vi "main_jgxu_double.vi"() -> ()   [LabVIEW 2012]
panel:
  out "Current-Time":cluster{dbl[], dbl[]}[](graph)
  in  "Quit":bool
  out "Voltage-Current":cluster{dbl[], dbl[]}[](graph)
  in  "Mode":enum32{"Main Panel", "0254 Initialize"}(tab)
  out "Boolean 2":bool
  in  "Start_2400":bool
  out "Time (s)":dbl
  in  "Delay (ms)":u32=1000
  in  "Target (V)":dbl=0.01
  in  "Step (V)":dbl=0.001
  in  "Stop":bool
  in  "file path (use dialog)":path=path "D:/TD/20171116/5-3/test.txt"
  in  "Ch1 Set":dbl=0.01
  out "Ch1 PV":dbl
  in  "Set Ch1":bool
  out "Boolean":bool
  out "SV_CH1":dbl
  in  "Ch2 Set Set":dbl=0.01
  out "SV_CH2":dbl
  out "Ch2 PV":dbl
  in  "Set Ch2":bool
  in  "VISA 2400":refnum<visa-resource-name>
  in  "VISA 0254":refnum<visa-resource-name>
  in  "Gas Flow Enable":bool
  in  "VISA 2450":refnum<visa-resource-name>
  in  "Target (V) Plas":dbl=0.01
  in  "Step (V) Plas":dbl=0.001
  in  "Initialization":bool
  out "Initiliazation Started":bool
  # "sccm"
  # "sccm"
  # "sccm"
  # "sccm"
  # "sccm"
  # "sccm"
  # "Please Wait  ~ 25 s"
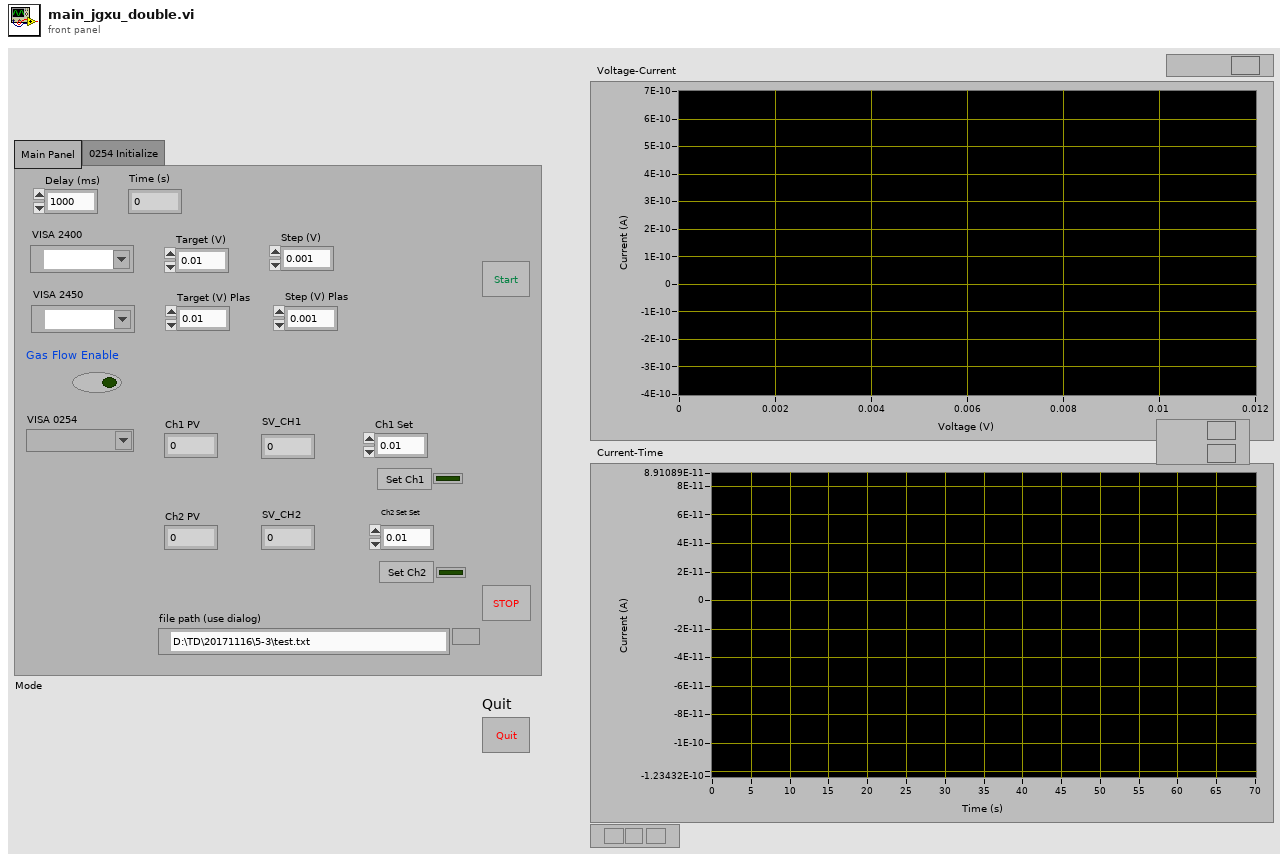
[diagram p1: front panel]
types:
  T1 = enum16{"open", "replace", "create", "open or create", "replace or create", "replace or create with confirmation"}
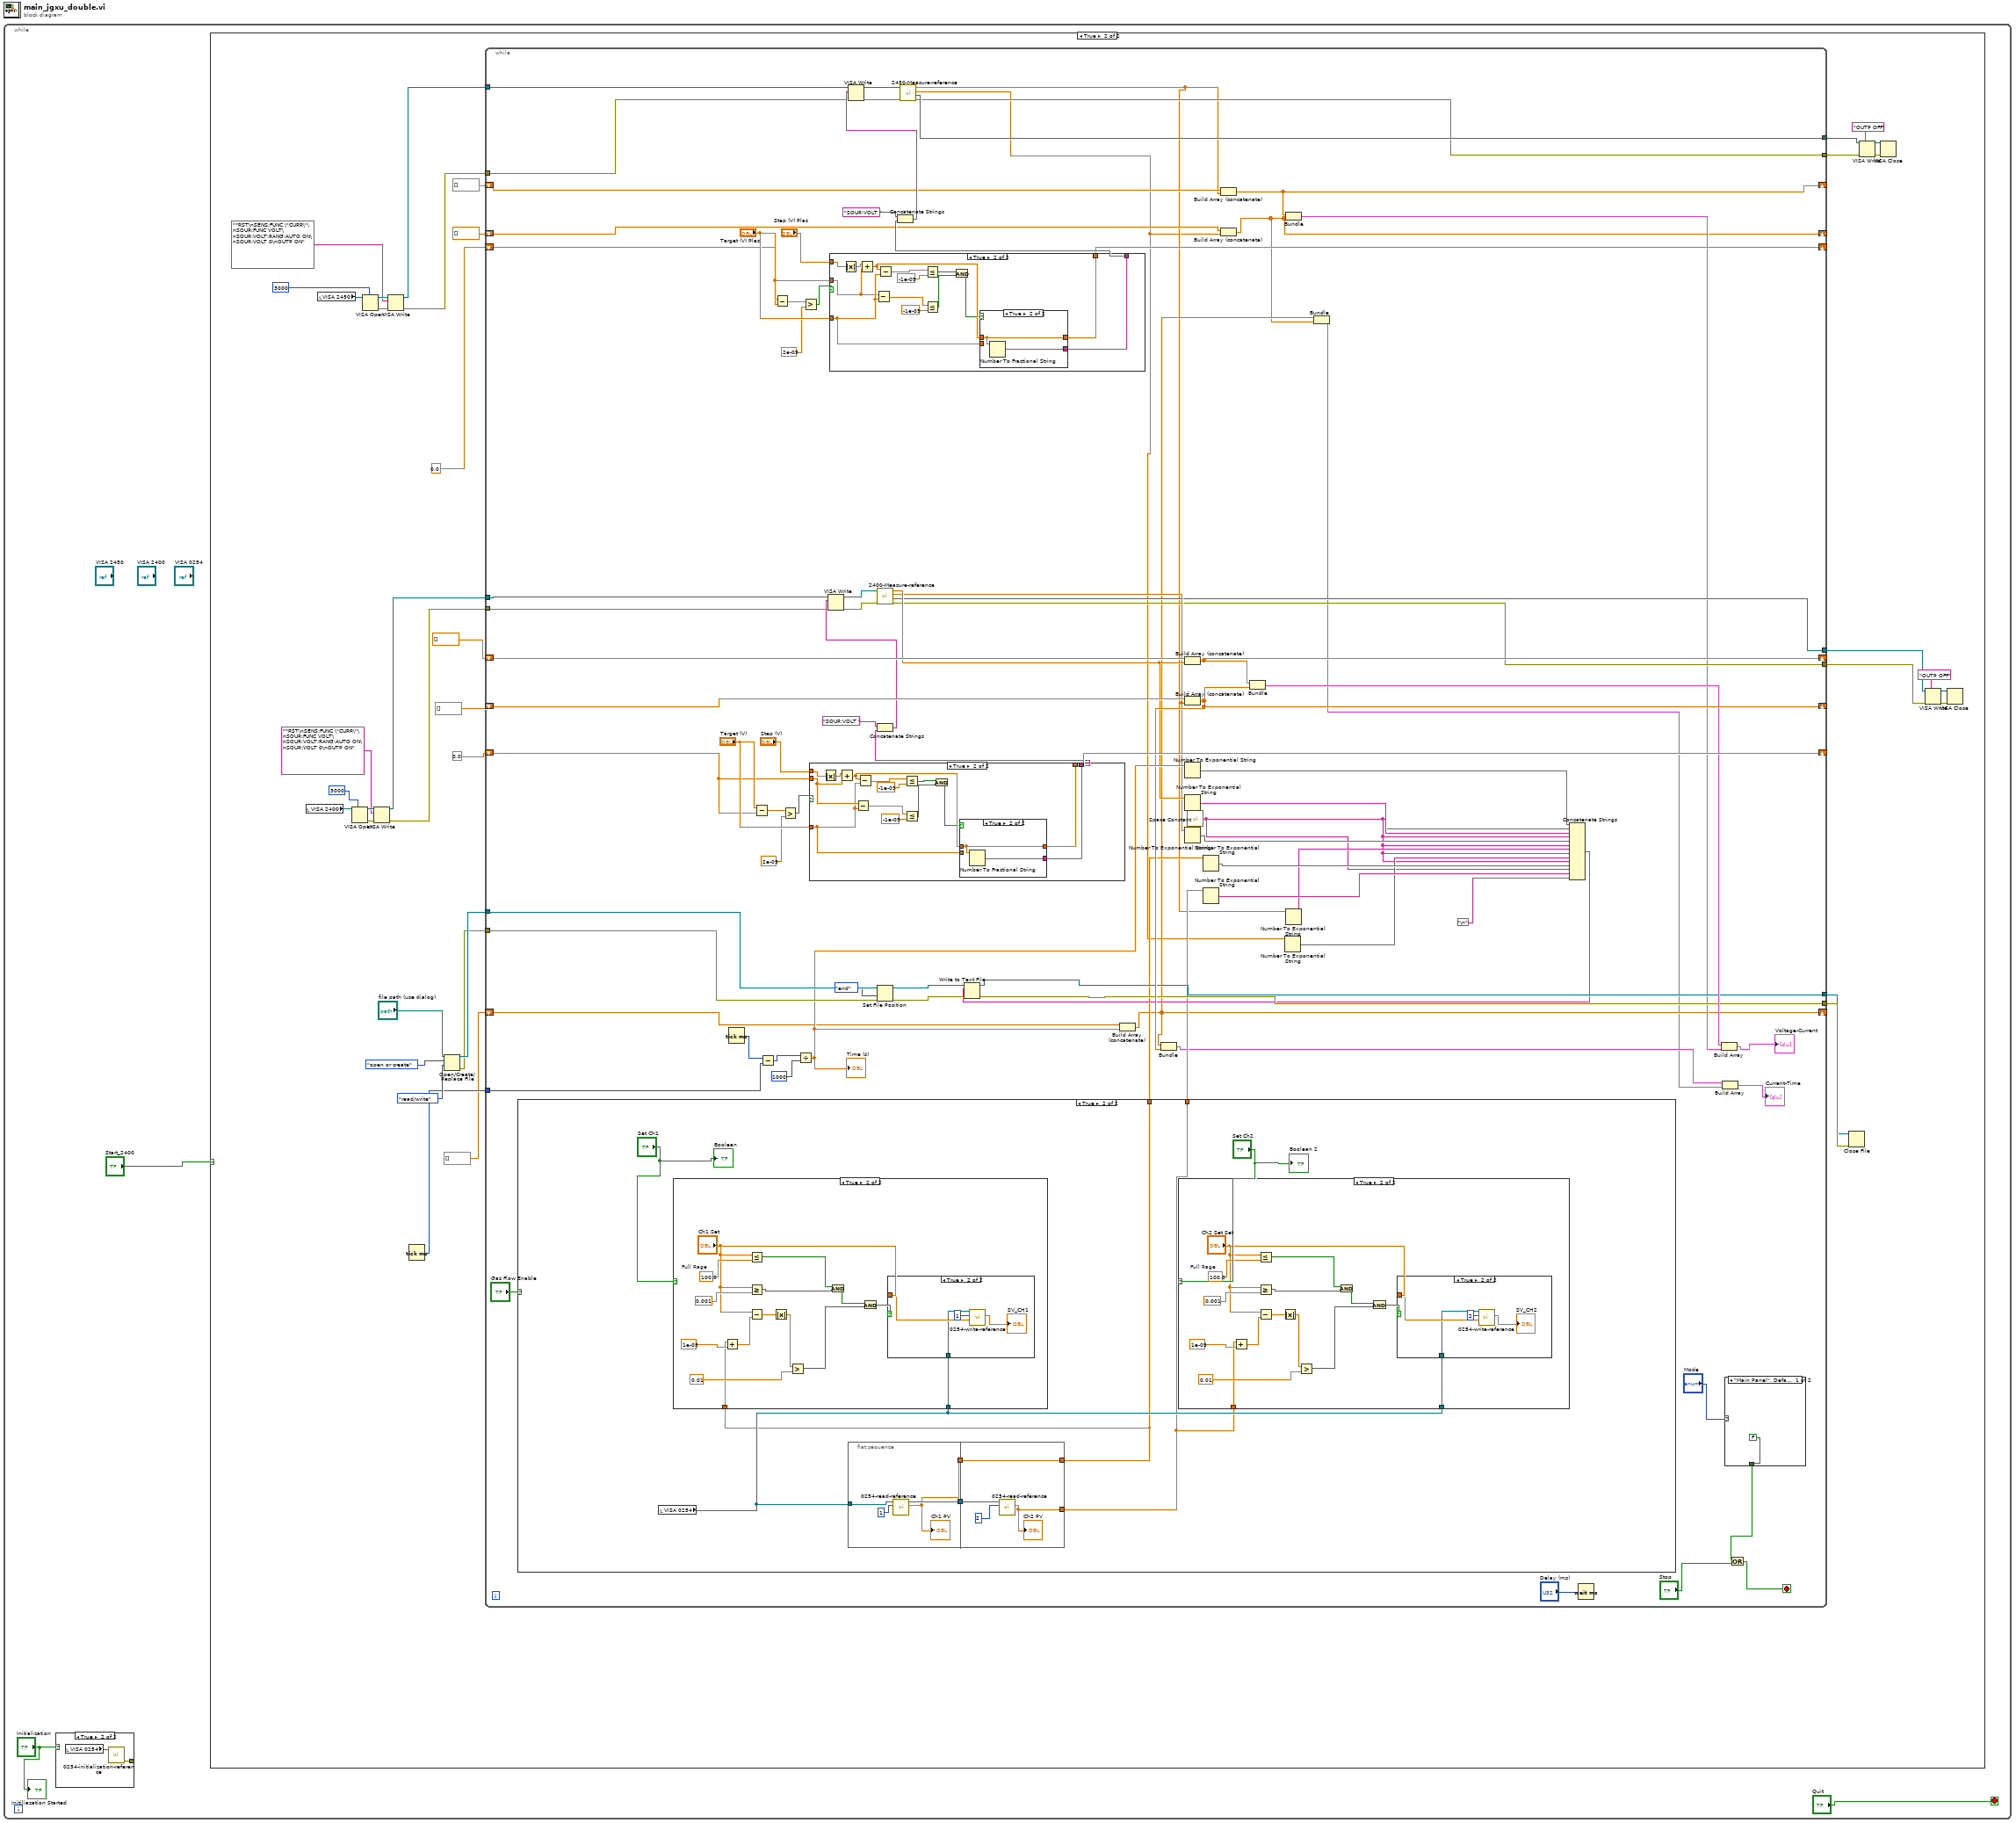
[diagram p0: block diagram]
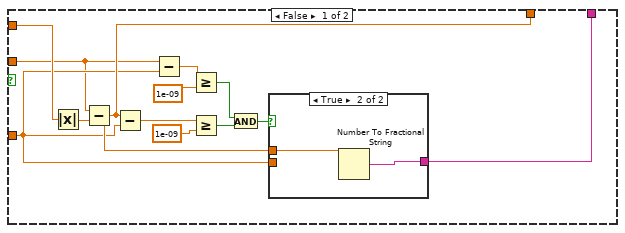
[diagram p3: hidden frame]
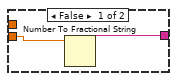
[diagram p4: hidden frame]
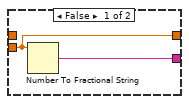
[diagram p5: hidden frame]
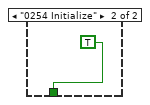
[diagram p6: hidden frame]
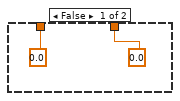
[diagram p7: hidden frame]
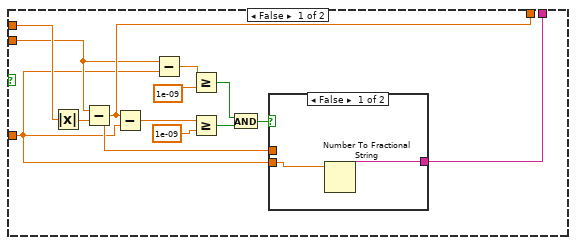
[diagram p12: hidden frame]
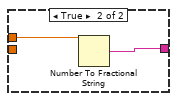
[diagram p13: hidden frame]
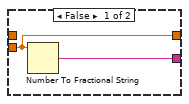
[diagram p14: hidden frame]
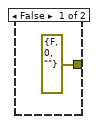
[diagram p15: hidden frame]
diagram:
  n1 = while {
    stop <- "Quit" stop-if-true
    n2 = case shown="True" "Initialization" {
      tunnel: [errorcluster {"status"=FALSE, "code"=0, "source"=""} ("error out") w253] -> _
      frame False {
      }
      frame True {
        n3 = local read "VISA 0254"() -> (w254:refnum<visa-resource-name>)
        n4 = call "0254-initialization-reference.vi"("0254-VISA"=w254) -> ("error out"=w253:errorcluster)  [unwired: 8 in, 2 out]
      }
    }
    n5 = case shown="True" "Start_2400" {
      frame False {
      }
      frame True {
        n6 = local read "VISA 2400"() -> (w28:refnum<visa-resource-name>)
        n7 = local read "VISA 2450"() -> (w15:refnum<visa-resource-name>)
        n8 = VISA Open(timeout (0)=3000 ("timeout ms (488.2 global)"), VISA resource name=w28) -> (VISA resource name=w31:refnum<visa-resource-name>, error out=w30:errorcluster)  [unwired: 3 in]
        n9 = VISA Open(timeout (0)=3000 ("timeout ms (488.2 global)"), VISA resource name=w15) -> (VISA resource name=w18:refnum<visa-resource-name>, error out=w17:errorcluster)  [unwired: 3 in]
        n10 = VISA Write(VISA resource name=w31, write buffer="*RST\nSENS:FUNC \"CURR\"\nSOUR:FUNC VOLT\nSOUR:VOLT:RANG:AUTO ON\nSOUR:VOLT 0\nOUTP ON" ("data"), error in (no error)=w30) -> (VISA resource name out=w25:refnum<visa-resource-name>, error out=w26:errorcluster)  [unwired: 1 out]
        n11 = VISA Write(VISA resource name=w18, write buffer="*RST\nSENS:FUNC \"CURR\"\nSOUR:FUNC VOLT\nSOUR:VOLT:RANG:AUTO ON\nSOUR:VOLT 0\nOUTP ON" ("data"), error in (no error)=w17) -> (VISA resource name out=w13:refnum<visa-resource-name>, error out=w12:errorcluster)  [unwired: 1 out]
        n12 = Tick Count (ms)() -> (millisecond timer value=w33:u32)
        n13 = Open/Create/Replace File(file path (use dialog)="file path (use dialog)", operation (0:open)=T1."open or create", access (0:read/write)=enum16{"read/write", "read-only", "write-only"}."read/write") -> (refnum out=w38:refnum<file>, error out=w37:errorcluster)  [unwired: 1 in, 3 out]
        n14 = while {
          shift-right: [w111] -> _
          shift-left: 0.0 ("Target (V)") -> [w107]
          shift-right: [w120] -> _
          shift-left: dbl[] [] -> [w123]
          shift-right: [w95] -> _
          shift-left: dbl[] [] -> [w122]
          tunnel: w38 -> [w117]
          tunnel: w37 -> [w116]
          tunnel: [w90] -> w36
          tunnel: [w91] -> w35
          tunnel: w25 -> [w103]
          tunnel: [w82] -> w21
          tunnel: [w81] -> w20
          tunnel: w26 -> [w94]
          tunnel: w33 -> [w101]
          shift-right: [w53] -> _
          shift-left: dbl[] [] -> [w96]
          tunnel: w13 -> [w65]
          tunnel: w12 -> [w64]
          shift-right: [w62] -> _
          shift-left: 0.0 ("Target (V)") -> [w63]
          tunnel: [w61] -> w7
          tunnel: [w60] -> w6
          shift-right: [w56] -> _
          shift-left: dbl[] [] -> [w57]
          shift-right: [w52] -> _
          shift-left: dbl[] [] -> [w55]
          stop <- w76 stop-if-true
          n15 = case shown="True" "Gas Flow Enable" {
            tunnel: [0.0 ("PV") w165] -> w88
            tunnel: [0.0 ("PV") w164] -> w87
            frame False {
            }
            frame True {
              n16 = local read "VISA 0254"() -> (w169:refnum<visa-resource-name>)
              n17 = case shown="True" "Set Ch1" {
                tunnel: w169 -> [_ w199]
                tunnel: w165 -> [_ w198]
                frame False {
                }
                frame True {
                  w202 = 100.0  # Full Rage
                  n18 = Add(x=w198, y=1e-05) -> (x+y=w211:dbl)
                  n19 = Less Or Equal?(x="Ch1 Set", y=w202) -> (x <= y?=w204:bool)
                  n20 = Greater Or Equal?(x="Ch1 Set", y=0.001) -> (x >= y?=w205:bool)
                  n21 = Subtract(x="Ch1 Set", y=w211) -> (x-y=w206:dbl)
                  n22 = Absolute Value(x=w206) -> (abs(x)=w207:dbl)
                  n23 = Greater?(x=w207, y=0.01) -> (0:w210:bool)
                  n24 = And(x=w204, y=w205) -> (x .and. y?=w209:bool)
                  n25 = And(x=w209, y=w210) -> (x .and. y?=w201:bool)
                  n26 = case shown="True" w201 {
                    tunnel: "Ch1 Set" -> [_ w216]
                    tunnel: w199 -> [_ w214]
                    frame False {
                    }
                    frame True {
                      n27 = call "0254-write-reference.vi"("SV"=w216, "Channel Selection"=1, "VISA Refnum in"=w214) -> ("SV_CH1"=→"SV_CH1":dbl)  [unwired: 6 in, 2 out]
                    }
                  }
                }
              }
              n28 = flat-sequence {
                tunnel: w169 -> [w173]
                tunnel: [w172] -> w167
                tunnel: [w171] -> w166
                tunnel: w167 -> [w177]
                tunnel: w166 -> [w176]
                tunnel: [w176] -> w165
                tunnel: [w175] -> w164
                frame #0 {
                  n29 = call "0254-read-reference.vi"("Channel Selction"=1, "VISA Refnum in"=w173) -> ("PV"=w171:dbl, "VISA Refnum out"=w172:refnum<visa-resource-name>)  [unwired: 7 in, 1 out]
                  "Ch1 PV" <- w171
                }
                frame #1 {
                  n30 = call "0254-read-reference.vi"("Channel Selction"=2 ("Channel Selction 2"), "VISA Refnum in"=w177) -> ("PV"=w175:dbl)  [unwired: 7 in, 2 out]
                  "Ch2 PV" <- w175
                }
              }
              n31 = case shown="True" "Set Ch2" {
                tunnel: w169 -> [_ w180]
                tunnel: w164 -> [_ w179]
                frame False {
                }
                frame True {
                  w183 = 100.0  # Full Rage
                  n32 = Add(x=w179, y=1e-05) -> (x+y=w192:dbl)
                  n33 = Less Or Equal?(x="Ch2 Set Set", y=w183) -> (x <= y?=w185:bool)
                  n34 = Greater Or Equal?(x="Ch2 Set Set", y=0.001) -> (x >= y?=w186:bool)
                  n35 = Subtract(x="Ch2 Set Set", y=w192) -> (x-y=w187:dbl)
                  n36 = Absolute Value(x=w187) -> (abs(x)=w188:dbl)
                  n37 = Greater?(x=w188, y=0.01) -> (0:w191:bool)
                  n38 = And(x=w185, y=w186) -> (x .and. y?=w190:bool)
                  n39 = And(x=w190, y=w191) -> (x .and. y?=w182:bool)
                  n40 = case shown="True" w182 {
                    tunnel: "Ch2 Set Set" -> [_ w197]
                    tunnel: w180 -> [_ w195]
                    frame False {
                    }
                    frame True {
                      n41 = call "0254-write-reference.vi"("SV"=w197, "Channel Selection"=2, "VISA Refnum in"=w195) -> ("SV_CH1"=→"SV_CH2":dbl)  [unwired: 6 in, 2 out]
                    }
                  }
                }
              }
              "Boolean" <- "Set Ch1"
              "Boolean 2" <- "Set Ch2"
            }
          }
          n42 = Tick Count (ms)() -> (millisecond timer value=w100:u32)
          n43 = Subtract(x="Target (V)", y=w107) -> (x-y=w106:dbl)
          n44 = Subtract(x=w100, y=w101) -> (x-y=w99:u32)
          n45 = Subtract(x="Target (V) Plas", y=w63) -> (x-y=w70:dbl)
          n46 = Greater?(x=w106, y=2e-09) -> (0:w110:bool)
          n47 = Divide(x=w99, y=u32 1000) -> (x/y=w97:dbl)
          "Time (s)" <- w97
          n48 = Greater?(x=w70, y=2e-09) -> (0:w73:bool)
          n49 = case shown="True" w110 {
            tunnel: "Step (V)" -> [w229 w247]
            tunnel: w107 -> [w224 w242]
            tunnel: "Target (V)" -> [w223 w241]
            tunnel: [w226 w244] -> w111
            tunnel: [w225 w243] -> w109
            frame False {
              n50 = Absolute Value(x=w229) -> (abs(x)=w228:dbl)
              n51 = Subtract(x=w224, y=w228) -> (x-y=w226:dbl)
              n52 = Subtract(x=w226, y=w223) -> (x-y=w218:dbl)
              n53 = Subtract(x=w224, y=w223) -> (x-y=w217:dbl)
              n54 = Greater Or Equal?(x=w217, y=1e-09) -> (x >= y?=w221:bool)
              n55 = Greater Or Equal?(x=w218, y=1e-09) -> (x >= y?=w220:bool)
              n56 = And(x=w221, y=w220) -> (x .and. y?=w219:bool)
              n57 = case shown="False" w219 {
                tunnel: w226 -> [_ w233]
                tunnel: [w230 w232] -> w225
                tunnel: w223 -> [w231 _]
                frame False {
                  n58 = Number To Fractional String(number=w231) -> (F-format string=w230:string)  [unwired: 3 in]
                }
                frame True {
                  n59 = Number To Fractional String(number=w233) -> (F-format string=w232:string)  [unwired: 3 in]
                }
              }
            }
            frame True {
              n60 = Absolute Value(x=w247) -> (abs(x)=w246:dbl)
              n61 = Add(x=w246, y=w242) -> (x+y=w245:dbl)
              n62 = Subtract(x=w242, y=w241) -> (x-y=w236:dbl)
              n63 = Subtract(x=w245, y=w241) -> (x-y=w239:dbl)
              n64 = Less Or Equal?(x=w239, y=-1e-09) -> (x <= y?=w237:bool)
              n65 = Less Or Equal?(x=w236, y=-1e-09) -> (x <= y?=w234:bool)
              n66 = And(x=w237, y=w234) -> (x .and. y?=w240:bool)
              n67 = case shown="True" w240 {
                tunnel: w245 -> [_ w250]
                tunnel: [w249 w251] -> w243
                tunnel: w241 -> [w248 _]
                tunnel: [w248 w250] -> w244
                frame False {
                  n68 = Number To Fractional String(number=w248) -> (F-format string=w249:string)  [unwired: 3 in]
                }
                frame True {
                  n69 = Number To Fractional String(number=w250) -> (F-format string=w251:string)  [unwired: 3 in]
                }
              }
            }
          }
          n70 = case shown="True" w73 {
            tunnel: "Step (V) Plas" -> [w137 w155]
            tunnel: "Target (V) Plas" -> [w132 w150]
            tunnel: [w134 w152] -> w62
            tunnel: [w133 w151] -> w72
            tunnel: w63 -> [w125 w142]
            frame False {
              n71 = Absolute Value(x=w137) -> (abs(x)=w136:dbl)
              n72 = Subtract(x=w125, y=w136) -> (x-y=w134:dbl)
              n73 = Subtract(x=w134, y=w132) -> (x-y=w127:dbl)
              n74 = Subtract(x=w125, y=w132) -> (x-y=w126:dbl)
              n75 = Greater Or Equal?(x=w126, y=1e-09) -> (x >= y?=w130:bool)
              n76 = Greater Or Equal?(x=w127, y=1e-09) -> (x >= y?=w129:bool)
              n77 = And(x=w130, y=w129) -> (x .and. y?=w128:bool)
              n78 = case shown="True" w128 {
                tunnel: w134 -> [_ w141]
                tunnel: [w138 w140] -> w133
                tunnel: w132 -> [w139 _]
                frame False {
                  n79 = Number To Fractional String(number=w139) -> (F-format string=w138:string)  [unwired: 3 in]
                }
                frame True {
                  n80 = Number To Fractional String(number=w141) -> (F-format string=w140:string)  [unwired: 3 in]
                }
              }
            }
            frame True {
              n81 = Absolute Value(x=w155) -> (abs(x)=w154:dbl)
              n82 = Add(x=w154, y=w142) -> (x+y=w153:dbl)
              n83 = Subtract(x=w142, y=w150) -> (x-y=w145:dbl)
              n84 = Subtract(x=w153, y=w150) -> (x-y=w148:dbl)
              n85 = Less Or Equal?(x=w148, y=-1e-09) -> (x <= y?=w146:bool)
              n86 = Less Or Equal?(x=w145, y=-1e-09) -> (x <= y?=w143:bool)
              n87 = And(x=w146, y=w143) -> (x .and. y?=w149:bool)
              n88 = case shown="True" w149 {
                tunnel: w153 -> [_ w158]
                tunnel: [w157 w159] -> w151
                tunnel: w150 -> [w156 _]
                tunnel: [w156 w158] -> w152
                frame False {
                  n89 = Number To Fractional String(number=w156) -> (F-format string=w157:string)  [unwired: 3 in]
                }
                frame True {
                  n90 = Number To Fractional String(number=w158) -> (F-format string=w159:string)  [unwired: 3 in]
                }
              }
            }
          }
          n91 = Concatenate Strings("SOUR:VOLT " ("string"), w109) -> (w104:string)
          n92 = VISA Write(VISA resource name=w103, write buffer=w104, error in (no error)=w94) -> (VISA resource name out=w86:refnum<visa-resource-name>, error out=w85:errorcluster)  [unwired: 1 out]
          n93 = Set File Position(refnum=w117, from (0:start)=enum16{"start", "end", "current"}."end", error in=w116) -> (refnum out=w115:refnum<file>, error out=w114:errorcluster)  [unwired: 1 out]
          n94 = call "2400-Measure-reference.vi"("error in (no error)"=w85, "VISA Refnum in"=w86) -> ("error out"=w81:errorcluster, "VISA resource name out"=w82:refnum<visa-resource-name>, "Current Output"=w83:dbl, "Voltage Output"=w84:dbl)  [unwired: 6 in]
          n95 = Concatenate Strings("SOUR:VOLT " ("string"), w72) -> (w68:string)
          n96 = VISA Write(VISA resource name=w65, write buffer=w68, error in (no error)=w64) -> (VISA resource name out=w67:refnum<visa-resource-name>, error out=w66:errorcluster)  [unwired: 1 out]
          n97 = call "2450-Measure-reference.vi"("error in (no error)"=w66, "VISA Refnum in"=w67) -> ("error out"=w60:errorcluster, "VISA resource name out"=w61:refnum<visa-resource-name>, "Current Output"=w46:dbl, "Voltage Output"=w47:dbl)  [unwired: 6 in]
          n98 = Build Array (concatenate)(w96, w97) -> (w53:dbl[])
          n99 = Build Array (concatenate)(w123, w84) -> (w120:dbl[])
          n100 = Build Array (concatenate)(w122, w83) -> (w95:dbl[])
          n101 = Bundle(w53, w95) -> (w59:cluster{dbl[], dbl[]})  [unwired: 1 in]
          n102 = Number To Exponential String(number=w97) -> (E-format string=w98:string)  [unwired: 3 in]
          n103 = Number To Exponential String(number=w84) -> (E-format string=w118:string)  [unwired: 3 in]
          n104 = Number To Exponential String(number=w83) -> (E-format string=w119:string)  [unwired: 3 in]
          n105 = call <vilib>:"Space Constant.vi"() -> ("String"=w43:string)
          n106 = Number To Exponential String(number=w88) -> (E-format string=w48:string)  [unwired: 3 in]
          n107 = Number To Exponential String(number=w87) -> (E-format string=w49:string)  [unwired: 3 in]
          n108 = Build Array (concatenate)(w57, w47) -> (w56:dbl[])
          n109 = Build Array (concatenate)(w55, w46) -> (w52:dbl[])
          n110 = Bundle(w120, w95) -> (w93:cluster{dbl[], dbl[]})  [unwired: 1 in]
          n111 = Number To Exponential String(number=w46) -> (E-format string=w44:string)  [unwired: 3 in]
          n112 = Number To Exponential String(number=w47) -> (E-format string=w45:string)  [unwired: 3 in]
          n113 = Bundle(w56, w52) -> (w54:cluster{dbl[], dbl[]})  [unwired: 1 in]
          n114 = Bundle(w53, w52) -> (w51:cluster{dbl[], dbl[]})  [unwired: 1 in]
          n115 = Concatenate Strings(w98, w43, w118, w43, w119, w43, w45, w43, w44, w43, w48, w43, w49, "\n") -> (w89:string)
          n116 = Write to Text File(file (use dialog)=w115, text=w89, error in=w114) -> (refnum out=w91:refnum<file>, error out=w90:errorcluster)  [unwired: 1 in, 1 out]
          n117 = Wait (ms)(milliseconds to wait="Delay (ms)") -> ()  [unwired: 1 out]
          n118 = Build Array(w93, w54) -> (→"Voltage-Current":cluster{dbl[], dbl[]}[])
          n119 = Build Array(w59, w51) -> (→"Current-Time":cluster{dbl[], dbl[]}[])
          n120 = case shown="\"Main Panel\", Default" "Mode" {
            tunnel: [FALSE TRUE] -> w78
            frame "Main Panel", Default {
            }
            frame "0254 Initialize" {
            }
          }
          n121 = Or(x=w78, y="Stop") -> (x .or. y?=w76:bool)
        }
        n122 = Close File(refnum=w35, error in=w36) -> ()  [unwired: 2 out]
        n123 = VISA Write(VISA resource name=w7, write buffer="OUTP OFF" ("data"), error in (no error)=w6) -> (VISA resource name out=w8:refnum<visa-resource-name>, error out=w9:errorcluster)  [unwired: 1 out]
        n124 = VISA Close(VISA resource name=w8, error in (no error)=w9) -> ()  [unwired: 1 out]
        n125 = VISA Write(VISA resource name=w21, write buffer="OUTP OFF" ("data"), error in (no error)=w20) -> (VISA resource name out=w23:refnum<visa-resource-name>, error out=w22:errorcluster)  [unwired: 1 out]
        n126 = VISA Close(VISA resource name=w23, error in (no error)=w22) -> ()  [unwired: 1 out]
      }
    }
    "Initiliazation Started" <- "Initialization"
  }
